vi "Destroy.vi"(0 "reference in":refnum<class "UUT.lvclass">, 5 "error in (no error)":errorcluster) -> (14 "reference out":refnum<class "UUT.lvclass">, 19 "error out":errorcluster)   [LabVIEW 2017, in "UUT.lvclass"]
uses:
  UUT.lvclass
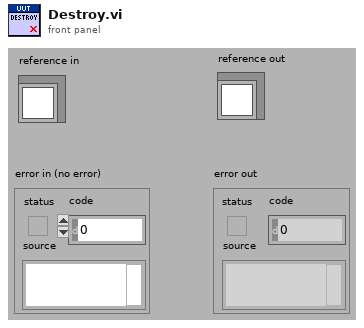
[diagram p1: front panel]
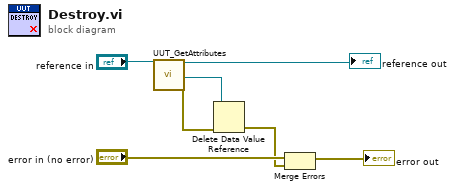
[diagram p0: block diagram]
diagram:
  n1 = call "UUT_GetAttributes.vi"("reference in"="reference in") -> ("reference out"=→"reference out":refnum<class "UUT.lvclass">, "DataRef"=w3:refnum<data-value>, "error out"=w4:errorcluster)  [unwired: 15 in, 1 out]
  n2 = Delete Data Value Reference(data value reference=w3, error in=w4) -> (error out=w1:errorcluster)  [unwired: 1 out]
  n3 = Merge Errors("error in (no error)", w1) -> (→"error out":errorcluster)
